vi "Timeout for Help2 Command-Default--Const.vi"() -> (3 "timeout (ms)":i32)   [LabVIEW 2017, in "Communications Library.lvlib"]
uses:
  Communications Library.lvlib
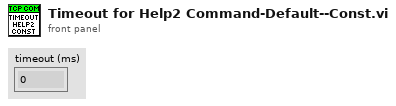
[diagram p1: front panel]
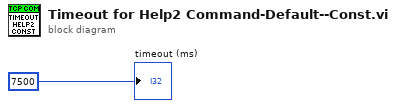
[diagram p0: block diagram]
diagram:
  "timeout (ms)" <- 7500 ("timeout ms (default 25000ms)")
